vi "Create TestRadio Object.vi"(10 "Position":u32, 11 "MTS Radio Test in":refnum<class "MTS Radio Test.lvclass">) -> (0 "error out":errorcluster, 3 "Test Radio out":refnum<class "SC Manufacturing Test.lvclass">)   [LabVIEW 2015, in "MTS Radio Test.lvclass"]
doc: "Creates and returns an NI-8452 device object."
uses:
  MTS Radio Test.lvclass
  Classes/Manufacturing Test/Class/SC Manufacturing Test.lvclass
  Classes/Test Recipe/Class/Test Recipe.lvclass
  Classes/Application/Class/Application.lvclass
  Test Class/Test Class.lvclass
  <vilib>/Cree, Inc/Cree Test Framework/Classes/Base Objects/Base Class/Base Class/Base Class.lvclass
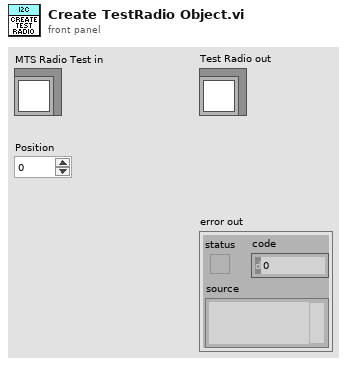
[diagram p1: front panel]
types:
  T1 = typedef "Application.lvlib/App Properties.lvclass/Class Properties -- Cluster.ctl" = cluster{"UUT Info":T2[], "Test Information":refnum<vi>, "Test Complete Event":refnum<user-event>, "Shop Floor System":refnum<class "Shop Floor System.lvclass">, "Gold Board":refnum<class "Golden Board.lvclass">, "Test Recipe":refnum<class "Test Recipe.lvclass">, "Instruments":refnum<class "Base Class.lvclass">[], "Mode":T3, "Test Results":cluster{"Pass":bool[], "Fail Codes":string[]}}
  T2 = typedef "Application.lvlib/App Properties.lvclass/UUT Reference -- Cluster.ctl" = cluster{"Serial Number Reference":refnum<vi>, "Status Message Reference":refnum<vi>}
  T3 = typedef "Application.lvlib/Application.lvclass/Op Mode -- Enum.ctl" = u16
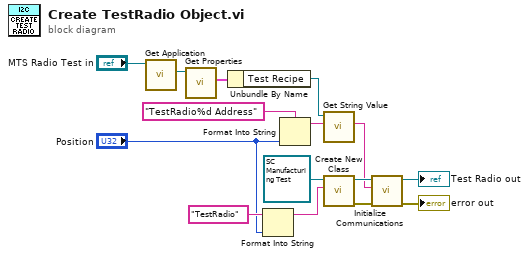
[diagram p0: block diagram]
diagram:
  n1 = call "Get Application.vi"("Test Class in"="MTS Radio Test in") -> ("Application.lvlib:Application.lvclass"=w13:refnum<class "Application.lvclass">)  [unwired: 9 in, 1 out]
  n2 = call "Get Properties.vi"("Acrobat Template in"=w13) -> ("Class Properties"=w12:T1)  [unwired: 8 in, 2 out]
  n3 = Unbundle By Name(w12) -> ("Test Recipe"=w14:refnum<class "Test Recipe.lvclass">)
  n4 = Format Into String(initial string="TestRadio" ("Name"), "Position") -> (resulting string=w2:string)  [unwired: 2 in, 1 out]
  n5 = Format Into String(format string="TestRadio%d Address" ("Name"), "Position") -> (resulting string=w11:string)  [unwired: 2 in, 1 out]
  n6 = call "Get String Value.vi"("Name"=w11, "Test Recipe in"=w14) -> ("Value"=w5:string)  [unwired: 7 in, 2 out]
  n7 = call <vilib>:"Create New Class.vi"("Name"=w2, "Base Class in"=refnum<class "SC Manufacturing Test.lvclass"> refnum ("SC Manufacturing Test in 2")) -> ("error out"=w7:errorcluster, "Base Class out"=w8:refnum<class "SC Manufacturing Test.lvclass">)  [unwired: 8 in]
  n8 = call "Initialize Communications.vi"("error in (no error)"=w7, "COM Port"=w5, "Acrobat Template in"=w8) -> ("error out"=→"error out":errorcluster, "Acrobat Template out"=→"Test Radio out":refnum<class "SC Manufacturing Test.lvclass">)  [unwired: 7 in]
